vi "Register Dynamic Events.vi"(8 "error in (no error)":errorcluster, 11 "IEventHandler In":refnum<class "IEventHandler.lvclass">) -> (0 "error out":errorcluster, 3 "IEventHandler Out":refnum<class "IEventHandler.lvclass">)   [LabVIEW 2020, in "MVA Framework.lvlib" / "ActorEvents.lvlib" / "IEventHandler.lvclass"]
doc: "抽象方法\n注册动态事件"
uses:
  IEventHandler.lvclass
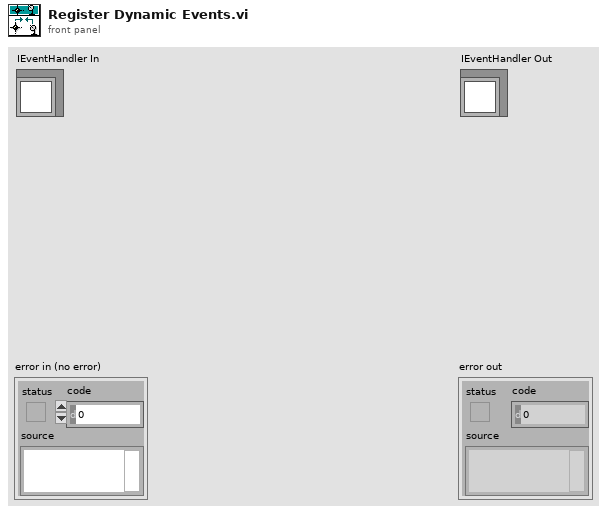
[diagram p1: front panel]
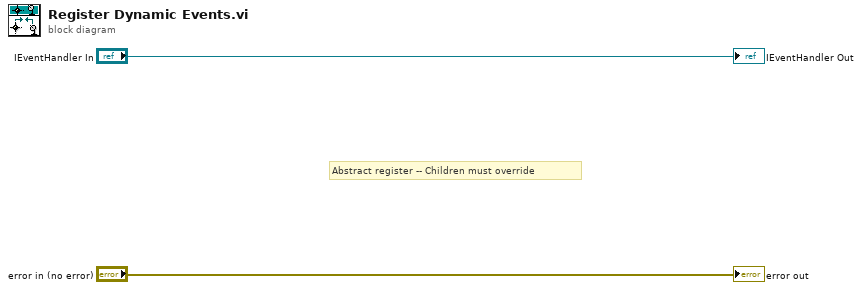
[diagram p0: block diagram]
diagram:
  # "Abstract register -- Children must override"
  "error out" <- "error in (no error)"
  "IEventHandler Out" <- "IEventHandler In"
